vi "RT_Control_Adrian_Microphones+Angles+Force.vi"(10 "rt fifo":refnum<k33>, 11 "Parameters":T1={"N_chan"=0, "Input Rate (Hz)"=0.0, "Acq Time (s)"=0.0, "NumOfWarmupIters"=0, "Size fifo"=0, "Period NCL (ms)"=0, "Timeout fifo Read"=0, "Size Sent Array"=0, "Output offsets"=[], "Input offsets"=[0.0, 0.0, 0.0, 0.0, 0.0, 0.0, 0.0, 0.0]}) -> (0 "error out":errorcluster, 1 "Total Iterations":i64, 2 "Delayed Cycles":dbl)   [LabVIEW 2021]
uses:
  parametersRT.ctl
  <vilib>/DAQmx/write.llb/DAQmx Write (Analog 1D DBL NChan 1Samp).vi
  <vilib>/DAQmx/read.llb/DAQmx Read (Analog 1D DBL NChan 1Samp).vi
  <vilib>/Analysis/baseanly.llb/A x Vector.vi
  <vilib>/DAQmx/read.llb/DAQmx Read (Digital 2D U32 NChan NSamp).vi
  <vilib>/Analysis/baseanly.llb/Mean (DBL).vi
  <vilib>/DAQmx/configure/timing.llb/DAQmx Timing (Sample Clock).vi
  <vilib>/DAQmx/miscellaneous.llb/DAQmx Fill In Error Info.vi
  <resource>/objmgr/daqmx.rc
  <vilib>/Analysis/NI_AALBase.lvlib
panel:
  out "subarray":dbl[](array[numeric])
  out "Power":dbl[](array[numeric])
  out "Current":dbl[](array[numeric])
  out "Voltages":dbl[](array[numeric])
  out "output array":dbl[](array[numeric])
  out "data 2":u32[][](array[numeric])
  out "Encoder Raw Outputs":dbl[][](array[numeric])
  out "Encoder Mean Outputs":dbl[](array[numeric])
  in  "Zero Angle":dbl[](array[numeric])=[-16.79, 2.64, -15.0, 3.7]
  in  "source 2":tag
  in  "source":tag
  out "A x Vector":dbl[](array[numeric]) format="%.2f"
  in  "Unbias":bool
  out "Bias Voltages":dbl[][](array[numeric])=[[-0.0710179470114859, -0.17463349299050945, -0.11016159714741332, 0.026018829634351103, 0.12897648926553976, 0.08259620236774425]]
  out "Bias Vector":dbl[](array[numeric])=[-0.0710179470114859, -0.17463349299050945, -0.11016159714741332, 0.026018829634351103, 0.12897648926553976, 0.08259620236774425]
  in  "Bias":bool
  out "Voltages":dbl[][](array[numeric])=[[-0.07200476171213811, -0.17430455474177844, -0.11114841186574954, 0.027005644288728526, 0.12535816905124034, 0.08062257311350753], [-0.07233369994578917, -0.17397561649309423, -0.11147735010529275, 0.027334582506747616, 0.1263449836558195, 0.08160938774087402], [-0.0716758234785372, -0.17463349299050945, -0.11147735010529275, 0.026676706070656076, 0.1260160454543497, 0.08062257311350753], [-0.07200476171213811, -0.1749624312392873, -0.1118062883448848, 0.026676706070656076, 0.1256871072528233, 0.08029363490427514], [-0.07200476171213811, -0.17430455474177844, -0.11213522658452575, 0.026676706070656076, 0.12535816905124034, 0.08029363490427514], [-0.07233369994578917, -0.1749624312392873, -0.11147735010529275, 0.027334582506747616, 0.1260160454543497, 0.08062257311350753], [-0.07200476171213811, -0.17397561649309423, -0.11147735010529275, 0.027005644288728526, 0.1260160454543497, 0.08029363490427514], [-0.07200476171213811, -0.17463349299050945, -0.1118062883448848, 0.027005644288728526, 0.1260160454543497, 0.08062257311350753], [-0.07233369994578917, -0.17397561649309423, -0.11114841186574954, 0.027334582506747616, 0.1263449836558195, 0.08062257311350753], [-0.07233369994578917, -0.17463349299050945, -0.1118062883448848, 0.026676706070656076, 0.1256871072528233, 0.08029363490427514], [-0.07200476171213811, -0.17463349299050945, -0.11213522658452575, 0.027334582506747616, 0.1256871072528233, 0.08062257311350753], [-0.07233369994578917, -0.17463349299050945, -0.1118062883448848, 0.027005644288728526, 0.1256871072528233, 0.08029363490427514], [-0.07200476171213811, -0.17463349299050945, -0.1118062883448848, 0.027334582506747616, 0.1260160454543497, 0.08029363490427514], [-0.0716758234785372, -0.17430455474177844, -0.11147735010529275, 0.027334582506747616, 0.1263449836558195, 0.08128044953180698], [-0.07200476171213811, -0.17463349299050945, -0.11114841186574954, 0.027005644288728526, 0.1263449836558195, 0.08029363490427514], [-0.07266263817949037, -0.17430455474177844, -0.11213522658452575, 0.027005644288728526, 0.1256871072528233, 0.08029363490427514], [-0.07233369994578917, -0.17463349299050945, -0.1118062883448848, 0.027334582506747616, 0.1263449836558195, 0.08128044953180698], [-0.07200476171213811, -0.17397561649309423, -0.1118062883448848, 0.026676706070656076, 0.1260160454543497, 0.08029363490427514], [-0.07233369994578917, -0.17397561649309423, -0.11147735010529275, 0.027334582506747616, 0.1263449836558195, 0.08128044953180698], [-0.0716758234785372, -0.17397561649309423, -0.11147735010529275, 0.027334582506747616, 0.1256871072528233, 0.08029363490427514], [-0.07200476171213811, -0.17430455474177844, -0.1118062883448848, 0.027334582506747616, 0.1263449836558195, 0.08095151132268481], [-0.07266263817949037, -0.17463349299050945, -0.1118062883448848, 0.026676706070656076, 0.1260160454543497, 0.08029363490427514], [-0.07200476171213811, -0.1736466782444569, -0.1118062883448848, 0.027005644288728526, 0.12535816905124034, 0.08095151132268481], [-0.07233369994578917, -0.1749624312392873, -0.11147735010529275, 0.027005644288728526, 0.1263449836558195, 0.08062257311350753], [-0.07200476171213811, -0.1736466782444569, -0.11114841186574954, 0.02766352072471333, 0.1263449836558195, 0.08062257311350753], [-0.07200476171213811, -0.17463349299050945, -0.1118062883448848, 0.027005644288728526, 0.1256871072528233, 0.08029363490427514], [-0.07266263817949037, -0.17430455474177844, -0.11213522658452575, 0.027334582506747616, 0.1260160454543497, 0.08062257311350753], [-0.07200476171213811, -0.17430455474177844, -0.11147735010529275, 0.02766352072471333, 0.1263449836558195, 0.08062257311350753], [-0.07200476171213811, -0.1749624312392873, -0.11213522658452575, 0.027334582506747616, 0.1260160454543497, 0.08062257311350753], [-0.07233369994578917, -0.17430455474177844, -0.11147735010529275, 0.027334582506747616, 0.1260160454543497, 0.08029363490427514], [-0.07233369994578917, -0.17397561649309423, -0.1118062883448848, 0.027334582506747616, 0.1263449836558195, 0.08062257311350753], [-0.0716758234785372, -0.17397561649309423, -0.11213522658452575, 0.027334582506747616, 0.1260160454543497, 0.07996469669498764], [-0.07266263817949037, -0.17430455474177844, -0.1118062883448848, 0.02766352072471333, 0.1263449836558195, 0.08062257311350753], [-0.07266263817949037, -0.17430455474177844, -0.1118062883448848, 0.027334582506747616, 0.1256871072528233, 0.08029363490427514], [-0.07200476171213811, -0.17463349299050945, -0.1118062883448848, 0.026676706070656076, 0.12535816905124034, 0.07963575848564507], [-0.07233369994578917, -0.17397561649309423, -0.11114841186574954, 0.02766352072471333, 0.1263449836558195, 0.08062257311350753], [-0.07266263817949037, -0.1749624312392873, -0.11213522658452575, 0.026676706070656076, 0.12535816905124034, 0.07963575848564507], [-0.07233369994578917, -0.17463349299050945, -0.1118062883448848, 0.027005644288728526, 0.1256871072528233, 0.07996469669498764], [-0.07299157641324171, -0.17463349299050945, -0.11213522658452575, 0.026676706070656076, 0.1260160454543497, 0.08029363490427514], [-0.07233369994578917, -0.17430455474177844, -0.11147735010529275, 0.027334582506747616, 0.12667392185723272, 0.08095151132268481], [-0.07200476171213811, -0.1736466782444569, -0.11147735010529275, 0.02766352072471333, 0.1263449836558195, 0.08062257311350753], [-0.07233369994578917, -0.17397561649309423, -0.1118062883448848, 0.026676706070656076, 0.1260160454543497, 0.07996469669498764], [-0.07233369994578917, -0.17463349299050945, -0.11213522658452575, 0.027005644288728526, 0.1260160454543497, 0.08029363490427514], [-0.07200476171213811, -0.17331773999586642, -0.11081947362625524, 0.02766352072471333, 0.12667392185723272, 0.08095151132268481], [-0.07233369994578917, -0.17397561649309423, -0.1118062883448848, 0.02766352072471333, 0.1260160454543497, 0.08029363490427514], [-0.07266263817949037, -0.17463349299050945, -0.11213522658452575, 0.02766352072471333, 0.1260160454543497, 0.08128044953180698], [-0.07200476171213811, -0.17397561649309423, -0.11147735010529275, 0.02766352072471333, 0.1263449836558195, 0.08095151132268481], [-0.07200476171213811, -0.17430455474177844, -0.1118062883448848, 0.027334582506747616, 0.1263449836558195, 0.08095151132268481], [-0.0716758234785372, -0.17463349299050945, -0.1118062883448848, 0.027005644288728526, 0.1263449836558195, 0.08095151132268481], [-0.07200476171213811, -0.17397561649309423, -0.1118062883448848, 0.027005644288728526, 0.1256871072528233, 0.08029363490427514], [-0.07233369994578917, -0.17430455474177844, -0.11147735010529275, 0.027334582506747616, 0.1263449836558195, 0.08095151132268481], [-0.0716758234785372, -0.1736466782444569, -0.11114841186574954, 0.027992458942625646, 0.12667392185723272, 0.08095151132268481], [-0.07200476171213811, -0.17397561649309423, -0.1118062883448848, 0.027334582506747616, 0.1263449836558195, 0.08029363490427514], [-0.07200476171213811, -0.17397561649309423, -0.11114841186574954, 0.027334582506747616, 0.1263449836558195, 0.08029363490427514], [-0.07233369994578917, -0.17397561649309423, -0.1118062883448848, 0.027334582506747616, 0.1260160454543497, 0.08029363490427514], [-0.07266263817949037, -0.17430455474177844, -0.11213522658452575, 0.026676706070656076, 0.1260160454543497, 0.08029363490427514], [-0.07233369994578917, -0.17397561649309423, -0.11213522658452575, 0.027334582506747616, 0.1263449836558195, 0.08062257311350753], [-0.07233369994578917, -0.17463349299050945, -0.11213522658452575, 0.027334582506747616, 0.1260160454543497, 0.08029363490427514], [-0.07200476171213811, -0.17331773999586642, -0.11147735010529275, 0.027334582506747616, 0.1263449836558195, 0.08029363490427514], [-0.07233369994578917, -0.1749624312392873, -0.11213522658452575, 0.026676706070656076, 0.1260160454543497, 0.08029363490427514], [-0.07233369994578917, -0.17463349299050945, -0.1118062883448848, 0.027005644288728526, 0.1260160454543497, 0.08029363490427514], [-0.07233369994578917, -0.17397561649309423, -0.1118062883448848, 0.027334582506747616, 0.12667392185723272, 0.08062257311350753], [-0.07200476171213811, -0.17430455474177844, -0.11147735010529275, 0.027334582506747616, 0.1260160454543497, 0.07996469669498764], [-0.07233369994578917, -0.17430455474177844, -0.1118062883448848, 0.027334582506747616, 0.12667392185723272, 0.08095151132268481], [-0.0716758234785372, -0.17430455474177844, -0.11147735010529275, 0.026676706070656076, 0.1263449836558195, 0.08029363490427514], [-0.07266263817949037, -0.17430455474177844, -0.11147735010529275, 0.027005644288728526, 0.1263449836558195, 0.07996469669498764], [-0.07266263817949037, -0.1749624312392873, -0.11246416482421552, 0.026676706070656076, 0.1263449836558195, 0.08029363490427514], [-0.07266263817949037, -0.17397561649309423, -0.1118062883448848, 0.027334582506747616, 0.1263449836558195, 0.08029363490427514], [-0.0716758234785372, -0.1736466782444569, -0.11147735010529275, 0.02766352072471333, 0.1263449836558195, 0.08062257311350753], [-0.07233369994578917, -0.17397561649309423, -0.1118062883448848, 0.027334582506747616, 0.1263449836558195, 0.08095151132268481], [-0.07233369994578917, -0.17430455474177844, -0.1118062883448848, 0.027334582506747616, 0.1260160454543497, 0.08062257311350753], [-0.0716758234785372, -0.17331773999586642, -0.11081947362625524, 0.027992458942625646, 0.12700286005858935, 0.08062257311350753], [-0.07233369994578917, -0.17397561649309423, -0.11213522658452575, 0.027005644288728526, 0.1263449836558195, 0.08029363490427514], [-0.07233369994578917, -0.17463349299050945, -0.11147735010529275, 0.027005644288728526, 0.1260160454543497, 0.08029363490427514], [-0.07266263817949037, -0.1736466782444569, -0.11147735010529275, 0.02766352072471333, 0.12667392185723272, 0.08029363490427514], [-0.07200476171213811, -0.17463349299050945, -0.11213522658452575, 0.026676706070656076, 0.1260160454543497, 0.07996469669498764], [-0.07266263817949037, -0.17430455474177844, -0.11213522658452575, 0.027005644288728526, 0.1263449836558195, 0.08062257311350753], [-0.07200476171213811, -0.17397561649309423, -0.11147735010529275, 0.02766352072471333, 0.1263449836558195, 0.08062257311350753], [-0.07200476171213811, -0.17397561649309423, -0.1118062883448848, 0.027005644288728526, 0.1263449836558195, 0.08029363490427514], [-0.07233369994578917, -0.17430455474177844, -0.11213522658452575, 0.027005644288728526, 0.1263449836558195, 0.08062257311350753], [-0.07233369994578917, -0.1736466782444569, -0.11114841186574954, 0.027334582506747616, 0.12667392185723272, 0.08062257311350753], [-0.07233369994578917, -0.17430455474177844, -0.1118062883448848, 0.027334582506747616, 0.1260160454543497, 0.08029363490427514], [-0.07266263817949037, -0.17529136948811197, -0.11279310306395414, 0.026676706070656076, 0.1263449836558195, 0.08029363490427514], [-0.07233369994578917, -0.17397561649309423, -0.11147735010529275, 0.027005644288728526, 0.12667392185723272, 0.08062257311350753], [-0.07200476171213811, -0.17430455474177844, -0.1118062883448848, 0.027334582506747616, 0.1263449836558195, 0.07996469669498764], [-0.07233369994578917, -0.17463349299050945, -0.11246416482421552, 0.027005644288728526, 0.1256871072528233, 0.07996469669498764], [-0.07266263817949037, -0.17430455474177844, -0.1118062883448848, 0.026676706070656076, 0.1260160454543497, 0.07996469669498764], [-0.07266263817949037, -0.17463349299050945, -0.1118062883448848, 0.027005644288728526, 0.1260160454543497, 0.08062257311350753], [-0.07266263817949037, -0.17397561649309423, -0.1118062883448848, 0.02766352072471333, 0.1263449836558195, 0.07996469669498764], [-0.07233369994578917, -0.17463349299050945, -0.1118062883448848, 0.027005644288728526, 0.1260160454543497, 0.08062257311350753], [-0.0716758234785372, -0.17397561649309423, -0.11114841186574954, 0.02766352072471333, 0.12667392185723272, 0.08095151132268481], [-0.07200476171213811, -0.17430455474177844, -0.11147735010529275, 0.027005644288728526, 0.1260160454543497, 0.08029363490427514], [-0.07200476171213811, -0.17397561649309423, -0.11114841186574954, 0.027992458942625646, 0.12700286005858935, 0.08128044953180698], [-0.07134688524498646, -0.17397561649309423, -0.1118062883448848, 0.027005644288728526, 0.1263449836558195, 0.07996469669498764], [-0.07266263817949037, -0.17463349299050945, -0.11213522658452575, 0.026676706070656076, 0.1256871072528233, 0.07996469669498764], [-0.07266263817949037, -0.17430455474177844, -0.11147735010529275, 0.027334582506747616, 0.12667392185723272, 0.08062257311350753], [-0.0716758234785372, -0.17463349299050945, -0.1118062883448848, 0.026676706070656076, 0.12667392185723272, 0.08029363490427514], [-0.07233369994578917, -0.17397561649309423, -0.1118062883448848, 0.027334582506747616, 0.1263449836558195, 0.08062257311350753], [-0.07233369994578917, -0.17463349299050945, -0.1118062883448848, 0.027005644288728526, 0.1260160454543497, 0.08029363490427514], [-0.07233369994578917, -0.17397561649309423, -0.11213522658452575, 0.027334582506747616, 0.1263449836558195, 0.08062257311350753]]
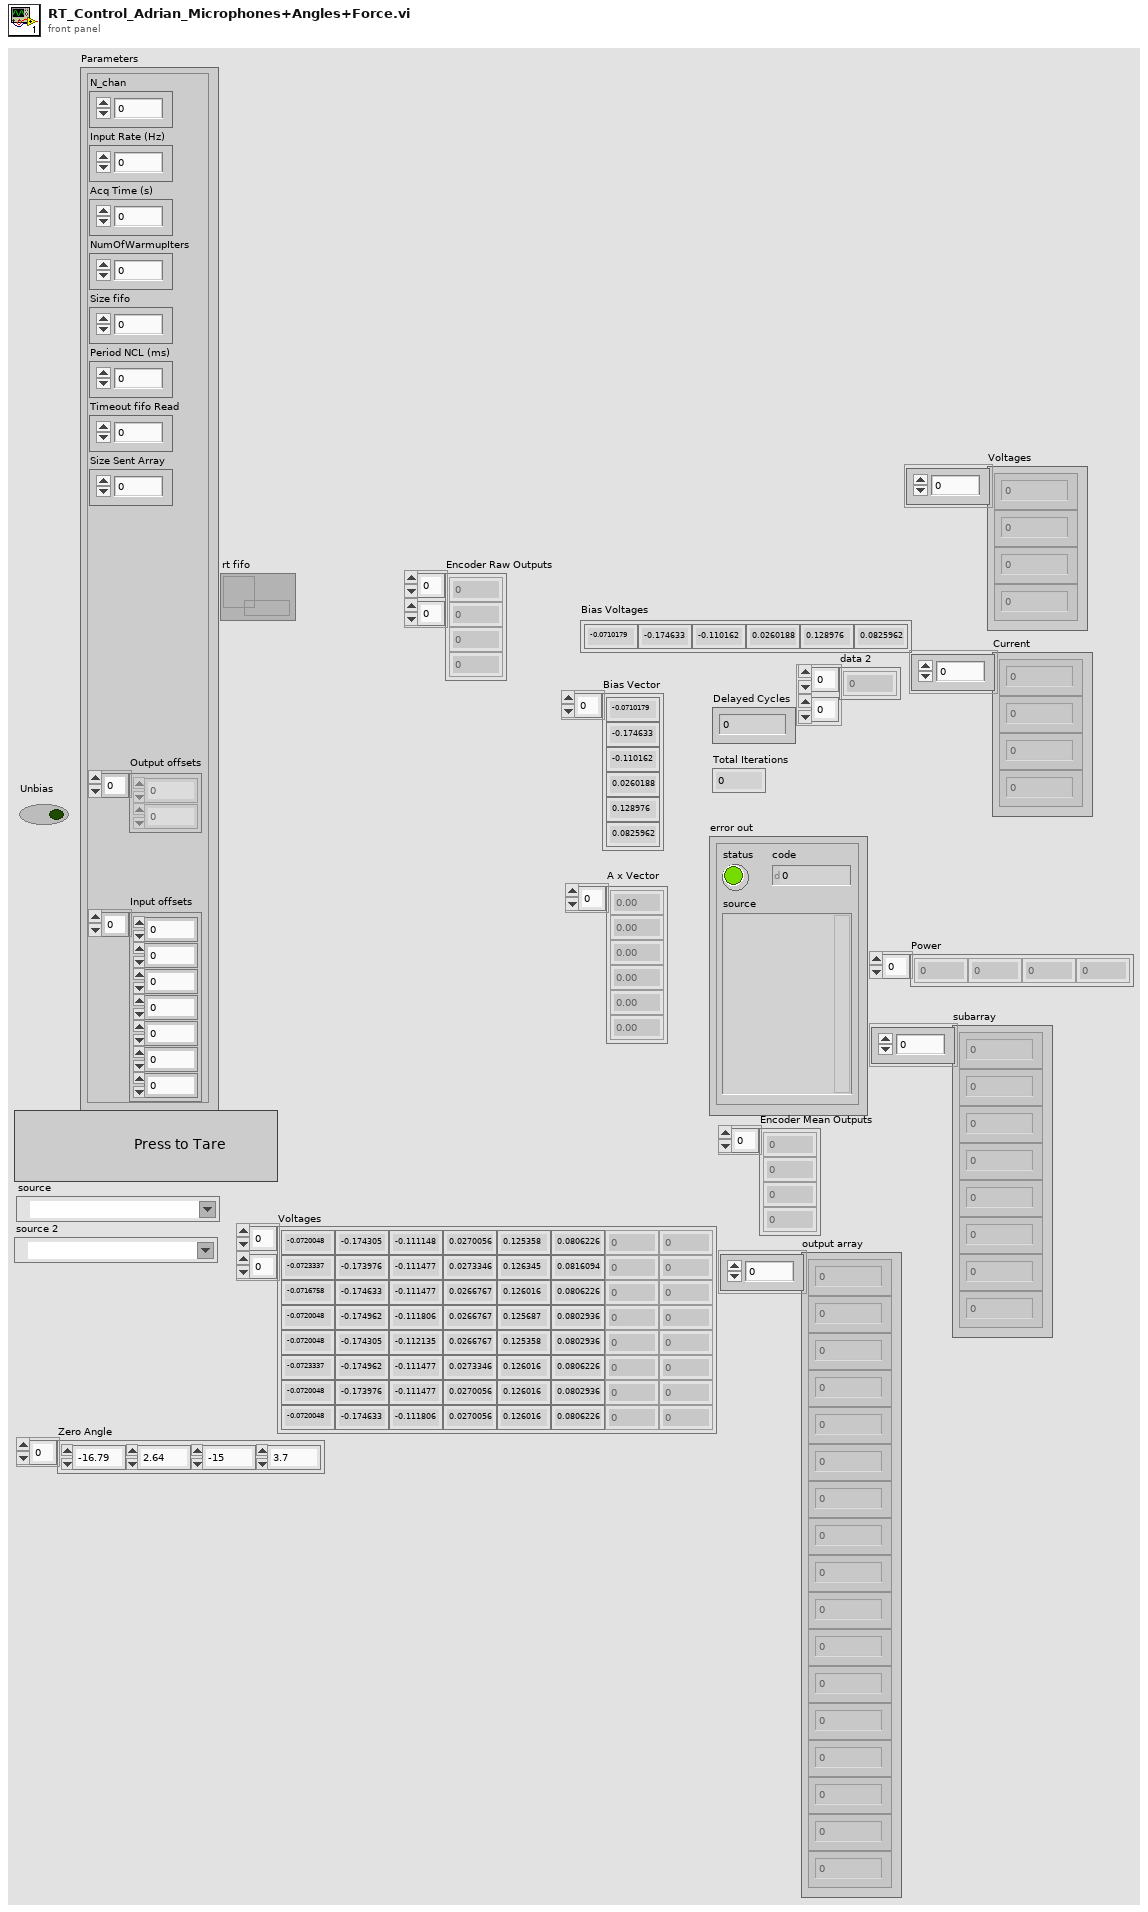
[diagram p1: front panel]
types:
  T1 = typedef "parametersRT.ctl" = cluster{"N_chan":u32, "Input Rate (Hz)":dbl, "Acq Time (s)":dbl, "NumOfWarmupIters":u32, "Size fifo":u32, "Period NCL (ms)":i64, "Timeout fifo Read":i32, "Size Sent Array":i32, "Output offsets":dbl[], "Input offsets":dbl[]}
  T2 = cluster{"Csn task out":refnum<k21>, "CLK task out":refnum<k21>, "D0 task out":refnum<k21>}
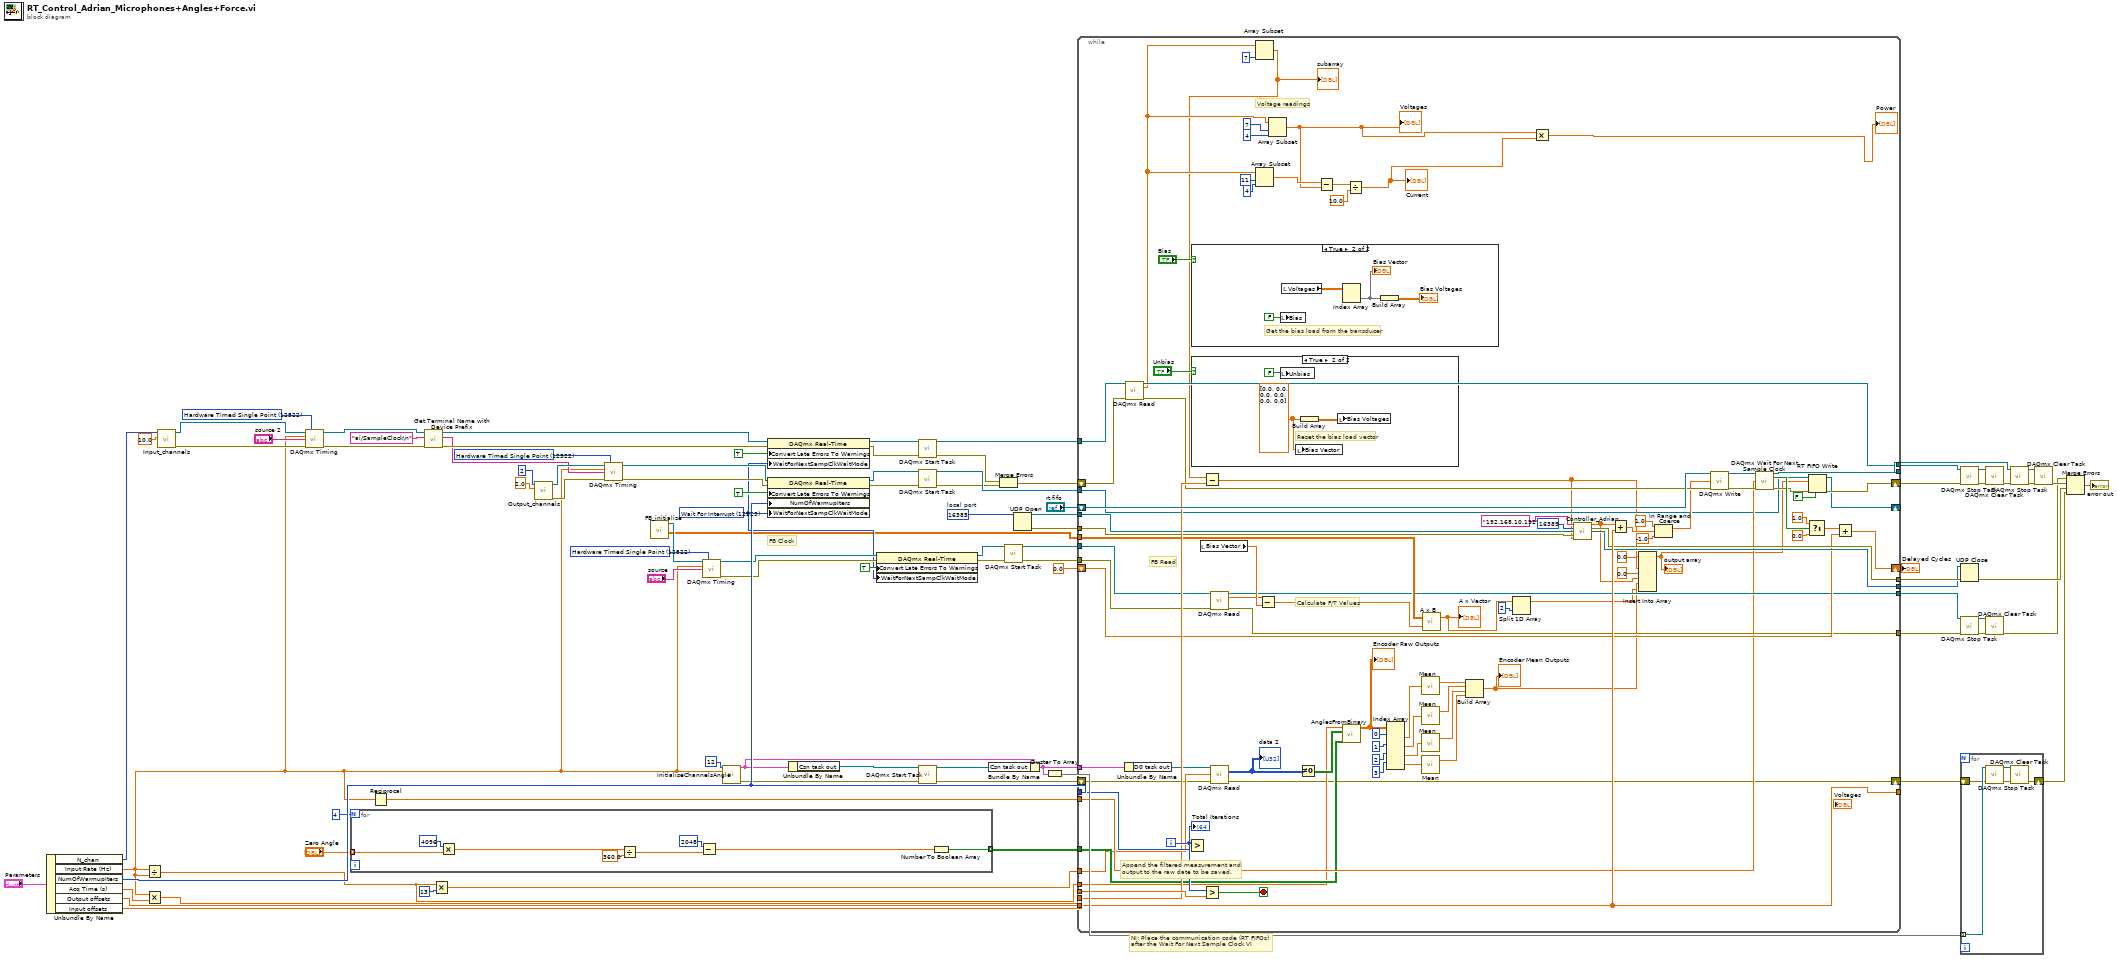
[diagram p0: block diagram]
diagram:
  w48 = 12522 items=["Finite Samples"=10178, "Continuous Samples"=10123, "Hardware Timed Single Point"=12522] ("sample mode")
  w59 = u16 16385  # local port
  w66 = 12522 items=["Finite Samples"=10178, "Continuous Samples"=10123, "Hardware Timed Single Point"=12522] ("sample mode")
  w43 = 12523 items=["Wait For Interrupt"=12523, "Poll"=12524, "Yield"=12525] ("WaitForNextSampClkWaitMode")
  w89 = 12522 items=["Finite Samples"=10178, "Continuous Samples"=10123, "Hardware Timed Single Point"=12522] ("sample mode")
  # "FB Clock"
  # "NI: Place the communication code (RT FIFOs) \nafter the Wait For Next Sample Clock VI"
  n1 = Unbundle By Name("Parameters") -> ("N_chan"=w75:u32, "Input Rate (Hz)"=w10:dbl, "NumOfWarmupIters"=w76:u32, "Acq Time (s)"=w83:dbl, "Output offsets"=w74:dbl[], "Input offsets"=w73:dbl[])
  n2 = Divide(x=w10, y=w10) -> (x/y=w8:dbl)
  n3 = Multiply(x=w10, y=w83) -> (x*y=w53:dbl)
  n4 = call "Input_channels.vi"("Range"=10.0, "nchan"=w75) -> ("error out"=w68:errorcluster, "Refnum out"=w67:refnum<k21>)  [unwired: 8 in]
  n5 = call-poly <vilib>:"DAQmx Timing.vi"("task/channels in"=w67, "sample mode"=w66, "rate"=w10, "source"="source 2", "error in"=w68) -> ("task out"=w36:refnum<k21>, "error out"=w34:errorcluster)  [unwired: 9 in]
  n6 = for {
    N: 4 -> [_]
    tunnel: [w94] -> w9 mode=indexing
    tunnel: "Zero Angle" -> [w97] mode=indexing
    n7 = Multiply(x=4096, y=w97) -> (x*y=w98:dbl)
    n8 = Divide(x=w98, y=360.0) -> (x/y=w92:dbl)
    n9 = Subtract(x=2048, y=w92) -> (x-y=w91:dbl)
    n10 = Number To Boolean Array(number=w91) -> (Boolean array=w94:bool[])
  }
  n11 = Reciprocal(x=w10) -> (1/x=w88:dbl)
  n12 = call "Get Terminal Name with Device Prefix.vi"("error in (no error)"=w34, "Local Terminal Name"="ai/SampleClock\n", "task/channels in"=w36) -> ("error out"=w33:errorcluster, "Terminal Name with Device Prefix"=w32:tag, "task out"=w35:refnum<k21>)  [unwired: 6 in]
  n13 = Multiply(x=w8, y=13) -> (x*y=w6:dbl)
  n14 = call "Output_channels.vi"("Range"=2.0 ("Maximum Value"), "nchan"=2) -> ("error out"=w80:errorcluster, "Refnum out"=w79:refnum<k21>)  [unwired: 8 in]
  n15 = call-poly <vilib>:"DAQmx Timing.vi"("task/channels in"=w79, "sample mode"=w89, "rate"=w10, "source"=w32, "error in"=w80) -> ("task out"=w87:refnum<k21>, "error out"=w86:errorcluster)  [unwired: 9 in]
  n16 = call "FB_initialize.vi"() -> ("Transformed Calibration Matrix"=w40:dbl[][], "FB out"=w44:refnum<k21>)  [unwired: 9 in, 1 out]
  n17 = call-poly <vilib>:"DAQmx Timing.vi"("task/channels in"=w44, "sample mode"=w48, "rate"=w10, "source"="source") -> ("task out"=w50:refnum<k21>, "error out"=w49:errorcluster)  [unwired: 10 in]
  n18 = call "InitialiseChannelsAngle.vi"("Number of data bits"=12, "Fs"=w10) -> ("output cluster"=w11:T2, "error out"=w12:errorcluster)  [unwired: 12 in]
  n19 = property class="DAQmx Real-Time"(reference=w35, error in=w33, "Convert Late Errors To Warnings"=TRUE, "WaitForNextSampClkWaitMode"=w43) -> (reference out=w63:refnum<k21>, error out=w62:errorcluster)
  n20 = property class="DAQmx Real-Time"(reference=w87, error in=w86, "Convert Late Errors To Warnings"=TRUE, "NumOfWarmupIters"=w76, "WaitForNextSampClkWaitMode"=w43) -> (reference out=w84:refnum<k21>, error out=w70:errorcluster)
  n21 = Unbundle By Name(w11) -> ("Csn task out"=w16:refnum<k21>)
  n22 = property class="DAQmx Real-Time"(reference=w50, error in=w49, "Convert Late Errors To Warnings"=TRUE ("ConvLateErrorsToWarnings"), "WaitForNextSampClkWaitMode"=w43) -> (reference out=w45:refnum<k21>, error out=w46:errorcluster)
  n23 = call <vilib>:"DAQmx Start Task.vi"("task/channels in"=w63, "error in"=w62) -> ("task out"=w82:refnum<k21>, "error out"=w61:errorcluster)  [unwired: 12 in]
  n24 = call <vilib>:"DAQmx Start Task.vi"("task/channels in"=w84, "error in"=w70) -> ("task out"=w81:refnum<k21>, "error out"=w69:errorcluster)  [unwired: 12 in]
  n25 = call <vilib>:"DAQmx Start Task.vi"("task/channels in"=w16, "error in"=w12) -> ("task out"=w15:refnum<k21>, "error out"=w3:errorcluster)  [unwired: 12 in]
  n26 = Bundle By Name(cluster=w11, "Csn task out"=w15) -> (w7:T2)
  n27 = Merge Errors(w61, w69) -> (w60:errorcluster)
  n28 = call <vilib>:"DAQmx Start Task.vi"("task/channels in"=w45, "error in"=w46) -> ("task out"=w42:refnum<k21>, "error out"=w41:errorcluster)  [unwired: 12 in]
  n29 = UDP Open(11:w59) -> (port=w57:refnum<k16>, 0:w58:errorcluster)  [unwired: 4 in, 1 out]
  n30 = Cluster To Array(cluster=w7) -> (array=w5:refnum<k21>[])
  n31 = while {
    shift-right: [w123] -> w25
    shift-left: w60 -> [w176]
    shift-right: [w185] -> w90
    shift-left: 0.0 ("f") -> [w164]
    tunnel: w88 -> [w147]
    tunnel: w53 -> [w183]
    tunnel: w81 -> [w182]
    tunnel: [w177] -> w24
    tunnel: w82 -> [w178]
    tunnel: [w149] -> w20
    tunnel: w76 -> [w180]
    tunnel: w74 -> [w172]
    tunnel: [w172] -> _
    tunnel: w73 -> [w179]
    tunnel: w58 -> [w170]
    tunnel: w57 -> [w169]
    tunnel: [w168] -> w56
    tunnel: [w167] -> w55
    tunnel: w42 -> [w163]
    tunnel: w41 -> [w162]
    tunnel: w40 -> [w157]
    tunnel: [w156] -> w30
    tunnel: [w155] -> w28
    tunnel: w9 -> [w130]
    tunnel: w8 -> [w129]
    tunnel: w7 -> [w128]
    tunnel: w6 -> [w127]
    shift-right: [w126] -> w4
    shift-left: w3 -> [w125]
    shift-right: [w115] -> _
    shift-left: "rt fifo" -> [w114]
    i -> [w181]
    stop <- w184 stop-if-true
    # "Voltage readings"
    # "Calculate F/T Values"
    # "FB Read"
    # "Append the filtered measurement and \noutput to the raw date to be saved."
    n32 = Unbundle By Name(w128) -> ("D0 task out"=w146:refnum<k21>)
    n33 = call-poly <vilib>:"DAQmx Read.vi"("task/channels in"=w178, "error in"=w176) -> ("task out"=w177:refnum<k21>, "data"=w104:dbl[], "error out"=w175:errorcluster)  [unwired: 11 in]
    n34 = Greater?(x=w181, y=w180) -> ()  [unwired: 1 out]
    n35 = case shown="True" "Bias" {
      frame False {
      }
      frame True {
        # "Get the bias load from the transducer"
        n36 = local write "Bias"(FALSE) -> ()
        n37 = local read "Voltages"() -> (w195:dbl[][])
        n38 = Index Array(array=w195) -> (element=w192:dbl[])  [unwired: 2 in]
        "Bias Vector" <- w192
        n39 = Build Array(w192) -> (→"Bias Voltages":dbl[][])
      }
    }
    n40 = case shown="True" "Unbias" {
      frame False {
      }
      frame True {
        w190 = dbl[] [0.0, 0.0, 0.0, 0.0, 0.0, 0.0]
        # "Reset the bias load vector"
        n41 = local write "Unbias"(FALSE) -> ()
        n42 = local write "Bias Vector"(w190) -> ()
        n43 = Build Array(w190) -> (w189:dbl[][])
        n44 = local write "Bias Voltages"(w189) -> ()
      }
    }
    n45 = local read "Bias Vector"() -> (w159:dbl[])
    n46 = Greater?(x=w181, y=w183) -> (0:w184:bool)
    n47 = call-poly <vilib>:"DAQmx Read.vi"("task/channels in"=w163, "error in"=w162) -> ("task out"=w156:refnum<k21>, "data"=w105:dbl[], "error out"=w155:errorcluster)  [unwired: 11 in]
    n48 = call-poly <vilib>:"DAQmx Read.vi"("task/channels in"=w146, "number of samples per channel"=w127, "error in"=w125) -> ("data"=w145:u32[][], "error out"=w126:errorcluster)  [unwired: 10 in, 1 out]
    "data 2" <- w145
    n49 = Array Subset(array=w104, length=7) -> (w103:dbl[])  [unwired: 1 in]
    "subarray" <- w103
    n50 = Subtract(x=w103, y=w179) -> (x-y=w99:dbl[])
    n51 = Array Subset(array=w104, index=11, length=4) -> (w106:dbl[])
    n52 = Subtract(x=w105, y=w159) -> (x-y=w158:dbl[])
    n53 = Array Subset(array=w104, index=7, length=4) -> (w102:dbl[])
    "Voltages" <- w102
    n54 = Not Equal To 0?(x=w145) -> (x != 0?=w131:bool[][])
    n55 = Subtract(x=w106, y=w102) -> (x-y=w108:dbl[])
    n56 = call "AnglesFromBinary.vi"("Binary Offset"=w130, "Array"=w131, "Buffer Length"=w129) -> ("Unwrapped Phase"=w144:dbl[][])  [unwired: 8 in]
    "Encoder Raw Outputs" <- w144
    n57 = Divide(x=w108, y=10.0) -> (x/y=w101:dbl[])
    "Current" <- w101
    n58 = Index Array(array=w144, index (row) #1=0 ("index (row)"), index (row) #2=1 ("index (row)"), index (row) #3=2 ("index (row)"), index (row) #4=3 ("index (row)")) -> (element #1=w139:dbl[], element #2=w138:dbl[], element #3=w137:dbl[], element #4=w136:dbl[])  [unwired: 4 in]
    n59 = call-poly <vilib>:"Mean.vi"("X"=w139) -> ("mean"=w132:dbl)  [unwired: 1 out]
    n60 = call-poly <vilib>:"Mean.vi"("X"=w138) -> ("mean"=w133:dbl)  [unwired: 1 out]
    n61 = call-poly <vilib>:"Mean.vi"("X"=w137) -> ("mean"=w134:dbl)  [unwired: 1 out]
    n62 = call-poly <vilib>:"Mean.vi"("X"=w136) -> ("mean"=w135:dbl)  [unwired: 1 out]
    n63 = call-poly <vilib>:"A x B.vi"("Vector"=w158, "A"=w157) -> ("A x Vector"=w153:dbl[])  [unwired: 1 out]
    "A x Vector" <- w153
    n64 = Build Array(w132, w133, w134, w135) -> (w118:dbl[])
    "Encoder Mean Outputs" <- w118
    n65 = Split 1D Array(array=w153, index=2) -> (first subarray=w117:dbl[])  [unwired: 1 out]
    n66 = Multiply(x=w102, y=w101) -> (x*y=→"Power":dbl[])
    n67 = call "Controller_Adrian.vi"("name 2"="192.168.10.192", "port or service name"=u16 16389, "connection ID"=w169, "error in (no error)"=w170, "x"=w99) -> ("*(type *) &x"=w119:dbl[], "error out"=w168:errorcluster, "connection ID out"=w167:refnum<k16>)  [unwired: 8 in]
    n68 = Add(x=w119, y=w172) -> (x+y=w152:dbl[])
    n69 = Insert Into Array(array=w99, new element #1=0.0 ("new element/subarray"), new element #2=0.0 ("new element/subarray"), new element #3=w119, new element #4=w118, new element #5=w117) -> (w116:dbl[])  [unwired: 1 in]
    "output array" <- w116
    n70 = In Range and Coerce(upper limit=1.0, x=w152, lower limit=-1.0) -> (coerced(x)=w171:dbl[])  [unwired: 1 out]
    n71 = call-poly <vilib>:"DAQmx Write.vi"("task/channels in"=w182, "data"=w171, "error in"=w175) -> ("task out"=w150:refnum<k21>, "error out"=w151:errorcluster)  [unwired: 10 in, 1 out]
    n72 = call <vilib>:"DAQmx Wait For Next Sample Clock.vi"("task/channels in"=w150, "timeout (sec)"=w147, "error in"=w151) -> ("task out"=w149:refnum<k21>, "is late?"=w148:bool, "error out"=w122:errorcluster)  [unwired: 10 in]
    n73 = Select(t=1.0, s=w148, f=0.0) -> (s? t:f=w186:dbl)
    n74 = RT FIFO Write(0:w114, 1:w116, 3:w122, 5:FALSE ("overwrite on timeout (T)")) -> (8:w115:refnum<k33>, 11:w123:errorcluster)  [unwired: 1 in, 2 out]
    n75 = Add(x=w186, y=w164) -> (x+y=w185:dbl)
    "Total Iterations" <- w181
  }
  "Delayed Cycles" <- w90
  n76 = call <vilib>:"DAQmx Stop Task.vi"("task/channels in"=w24, "error in"=w25) -> ("task out"=w23:refnum<k21>, "error out"=w26:errorcluster)  [unwired: 12 in]
  n77 = UDP Close(connection ID=w55, 8:w56) -> (error out=w54:errorcluster)  [unwired: 1 out]
  n78 = call <vilib>:"DAQmx Stop Task.vi"("task/channels in"=w30, "error in"=w28) -> ("task out"=w29:refnum<k21>, "error out"=w27:errorcluster)  [unwired: 12 in]
  n79 = for {
    tunnel: w5 -> [w200] mode=indexing
    shift-right: [w196] -> w2
    shift-left: w4 -> [w198]
    n80 = call <vilib>:"DAQmx Stop Task.vi"("task/channels in"=w200, "error in"=w198) -> ("task out"=w199:refnum<k21>, "error out"=w197:errorcluster)  [unwired: 12 in]
    n81 = call <vilib>:"DAQmx Clear Task.vi"("task in"=w199, "error in"=w197) -> ("error out"=w196:errorcluster)  [unwired: 13 in]
  }
  n82 = call <vilib>:"DAQmx Clear Task.vi"("task in"=w23, "error in"=w26) -> ("error out"=w22:errorcluster)  [unwired: 13 in]
  n83 = call <vilib>:"DAQmx Clear Task.vi"("task in"=w29, "error in"=w27) -> ("error out"=w39:errorcluster)  [unwired: 13 in]
  n84 = call <vilib>:"DAQmx Stop Task.vi"("task/channels in"=w20, "error in"=w22) -> ("task out"=w19:refnum<k21>, "error out"=w21:errorcluster)  [unwired: 12 in]
  n85 = call <vilib>:"DAQmx Clear Task.vi"("task in"=w19, "error in"=w21) -> ("error out"=w72:errorcluster)  [unwired: 13 in]
  n86 = Merge Errors(w39, w72, w54, w2) -> (→"error out":errorcluster)
